vi "Get Nth Element.vi"(10 "index":i32, 11 "Ordered Array.lvclass in":refnum<class "Ordered Array.lvclass">) -> (2 "Element":u32, 3 "Ordered Array.lvclass out":refnum<class "Ordered Array.lvclass">)   [LabVIEW 2011, in "Ordered Array.lvclass"]
uses:
  Ordered Array.lvclass
  Ordered Array.lvclass/Ordered Array.ctl
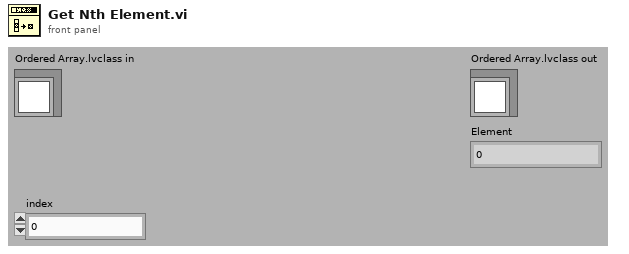
[diagram p1: front panel]
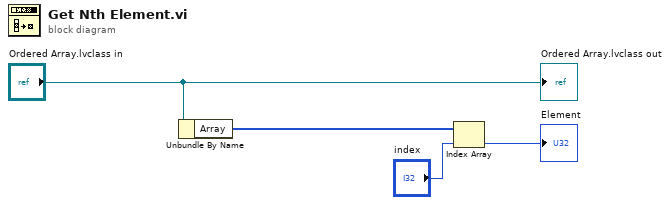
[diagram p0: block diagram]
diagram:
  n1 = Unbundle By Name("Ordered Array.lvclass in") -> ("Array"=w2:u32[])
  n2 = Index Array(array=w2, index="index") -> (element=→"Element":u32)
  "Ordered Array.lvclass out" <- "Ordered Array.lvclass in"
